vi "ClassItems.vi"(11 "ProjectItem in":refnum<vi>) -> (3 "Owned Items[]":refnum<vi>[](array[refnum]))   [LabVIEW 2021, in "Tree.lvlib" / "Tree.lvclass"]
uses:
  Tree.lvclass
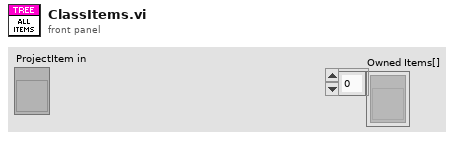
[diagram p1: front panel]
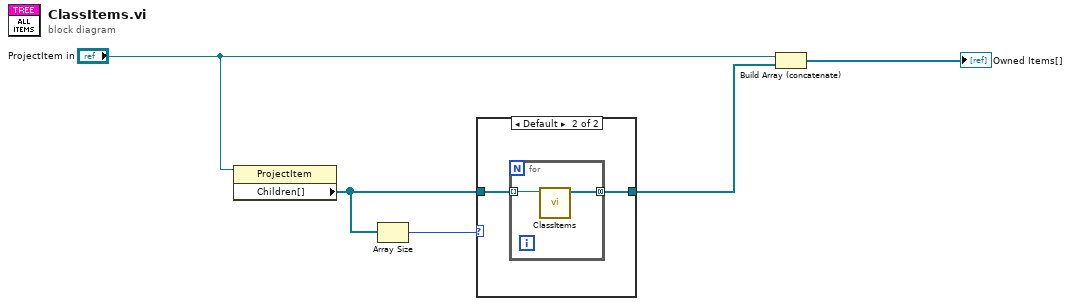
[diagram p0: block diagram]
diagram:
  n1 = property class="ProjectItem"(reference="ProjectItem in") -> ("Children[]"=w2:refnum<vi>[])  [unwired: 1 in, 2 out]
  n2 = Array Size(array=w2) -> (size(s)=w1:i32)
  n3 = case shown="Default" w1 {
    tunnel: [_ w7] -> w3
    tunnel: w2 -> [_ w6]
    frame 0 {
    }
    frame Default {
      n4 = for {
        tunnel: w6 -> [w9] mode=indexing
        tunnel: [w8] -> w7 mode=concatenating
        n5 = call "ClassItems.vi"("ProjectItem in"=w9) -> ("Owned Items[]"=w8:refnum<vi>[])  [unwired: 10 in]
      }
    }
  }
  n6 = Build Array (concatenate)("ProjectItem in", w3) -> (→"Owned Items[]":refnum<vi>[])
